vi "Get Multi.vi"(0 "Display State In":T1={"mixed"=FALSE, "format"="%#g", "Value"=0.0}, 7 "Value In":dbl, 9 "Container State":T2, 11 "error in (no error)":errorcluster) -> (4 "Display State Out":T1={"mixed"=FALSE, "format"="%#g", "Value"=0.0}, 8 "Value Out":dbl, 15 "error out":errorcluster)   [LabVIEW 2015, in "KNumeric (DBL).xctl"]
uses:
  KNumeric (DBL).xctl
  <vilib>/_xctls/Container State.ctl
  State.ctl
  <vilib>/_xctls/XControlSupport.lvlib
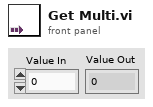
[diagram p1: front panel]
types:
  T1 = typedef "KNumeric (DBL).xctl/State.ctl" = cluster{"mixed":bool, "format":string, "Value":dbl}
  T2 = typedef "XControlSupport.lvlib/Container State.ctl" = cluster{"Indicator?":bool, "Run Mode?":bool, " Refnum":refnum<vi>}
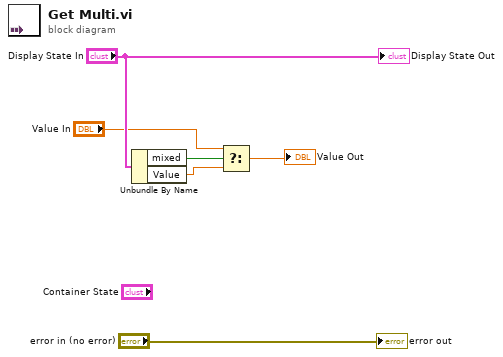
[diagram p0: block diagram]
diagram:
  n1 = Unbundle By Name("Display State In") -> ("mixed"=w4:bool, "Value"=w1:dbl)
  n2 = Select(t="Value In", s=w4, f=w1) -> (s? t:f=→"Value Out":dbl)
  "Display State Out" <- "Display State In"
  "error out" <- "error in (no error)"
